vi "SAOMM-SetROIProperties.vi"(0 "PRAMMS-COMM IN":refnum<visa-resource-name>="COM4", 1 "Active Refnum":refnum<vi>, 2 "ACK Refnum":refnum<vi>, 3 "MessageType":cluster{string[], u32[]}, 11 "Error IN":errorcluster, 13 "ROIProperties":T1) -> (4 "PRAMMS-COMM OUT":refnum<visa-resource-name>="COM4", 8 "Error":bool, 15 "Error OUT":errorcluster)   [LabVIEW 2011]
panel:
  out "Array":u32[](array[numeric])
  in  "Signature":u32=1886544237
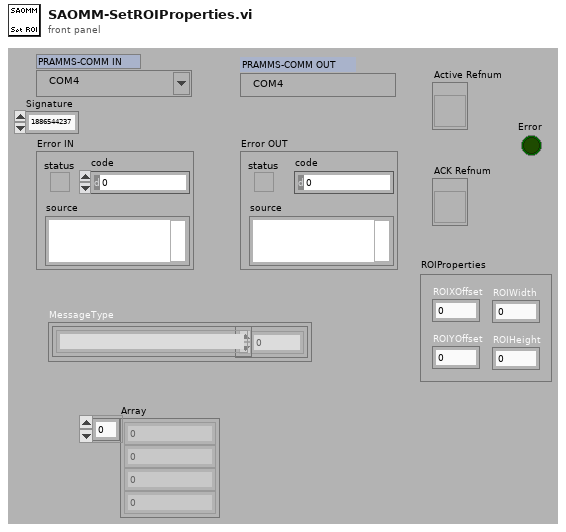
[diagram p1: front panel]
types:
  T1 = cluster{"ROIXOffset":u16, "ROIYOffset":u16, "ROIWidth":u16, "ROIHeight":u16}
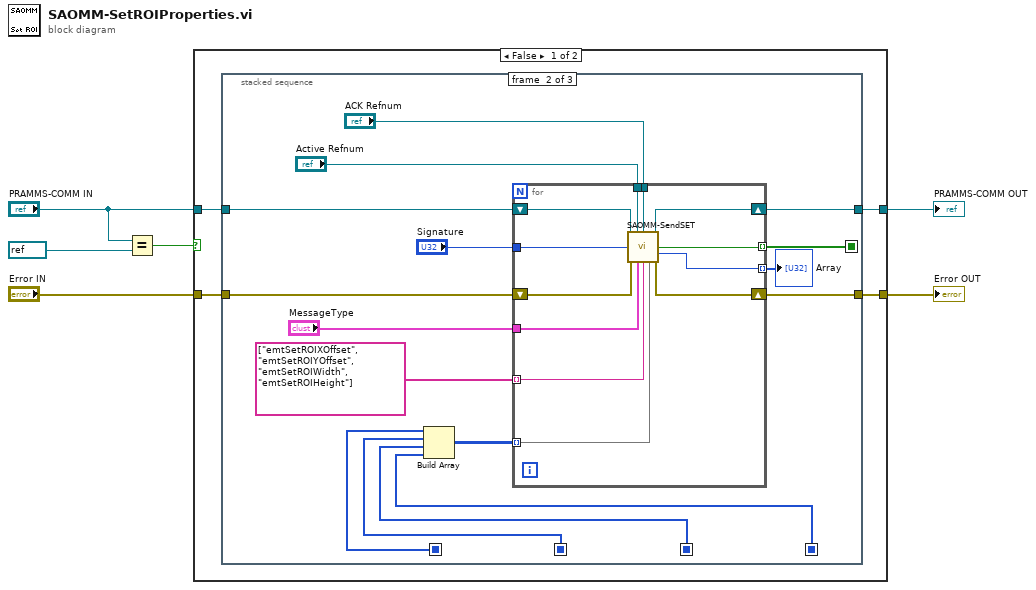
[diagram p0: block diagram]
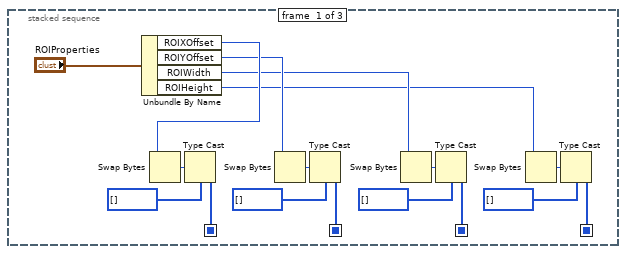
[diagram p2: hidden frame]
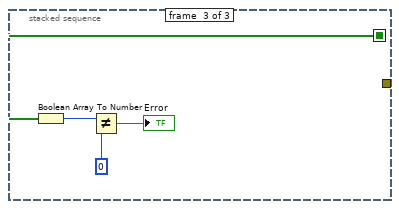
[diagram p3: hidden frame]
diagram:
  n1 = Equal?(x="PRAMMS-COMM IN", y=refnum<visa-resource-name> "-1") -> (x = y?=w5:bool)
  n2 = case shown="False" w5 {
    tunnel: "PRAMMS-COMM IN" -> [w10 w61]
    tunnel: "Error IN" -> [w9 w60]
    tunnel: [w8 w61] -> w2
    tunnel: [w7 w60] -> w1
    frame False {
      n3 = stacked-sequence {
        seq-local: [w19 _ _] -> [_ w40 _]
        seq-local: [w18 _ _] -> [_ w41 _]
        seq-local: [w17 _ _] -> [_ w42 _]
        seq-local: [w16 _ _] -> [_ w43 _]
        seq-local: [_ w31 _] -> [_ _ w59]
        tunnel: w10 -> [_ w38 _]
        tunnel: w9 -> [_ w37 _]
        tunnel: [_ w36 _] -> w8
        tunnel: [_ w35 _] -> w7
        frame #0 {
          n4 = Unbundle By Name("ROIProperties") -> ("ROIXOffset"=w14:u16, "ROIYOffset"=w13:u16, "ROIWidth"=w12:u16, "ROIHeight"=w11:u16)
          n5 = Swap Bytes(anything=w14) -> (byte swapped=w26:u16)
          n6 = Type Cast(type=u8[] [] ("Value (little endianed byte array)"), x=w26) -> (*(type *) &x=w19:u8[])
          n7 = Swap Bytes(anything=w13) -> (byte swapped=w25:u16)
          n8 = Type Cast(type=u8[] [] ("Value (little endianed byte array)"), x=w25) -> (*(type *) &x=w18:u8[])
          n9 = Swap Bytes(anything=w12) -> (byte swapped=w22:u16)
          n10 = Type Cast(type=u8[] [] ("Value (little endianed byte array)"), x=w22) -> (*(type *) &x=w17:u8[])
          n11 = Swap Bytes(anything=w11) -> (byte swapped=w21:u16)
          n12 = Type Cast(type=u8[] [] ("Value (little endianed byte array)"), x=w21) -> (*(type *) &x=w16:u8[])
        }
        frame #1 {
          n13 = Build Array(w40, w41, w42, w43) -> (w39:u8[][])
          n14 = for {
            tunnel: w39 -> [w48] mode=indexing
            shift-right: [w53] -> w36
            shift-left: w38 -> [w54]
            shift-right: [w52] -> w35
            shift-left: w37 -> [w55]
            tunnel: string[] ["emtSetROIXOffset", "emtSetROIYOffset", "emtSetROIWidth", "emtSetROIHeight"] -> [w49] mode=indexing
            tunnel: "ACK Refnum" -> [w50]
            tunnel: "Active Refnum" -> [w51]
            tunnel: [w47] -> w31 mode=indexing
            tunnel: "MessageType" -> [w46]
            tunnel: "Signature" -> [w45]
            tunnel: [w44] -> w28 mode=indexing
            n15 = call "SAOMM-SendSET.vi"("PRAMMS-COMM IN"=w54, "Active Refnum"=w51, "ACK Refnum"=w50, "Signature"=w45, "Error IN"=w55, "MessageType"=w46, "Active SET"=w49, "Value (little endianed byte array)"=w48) -> ("PRAMMS-COMM OUT"=w53:refnum<visa-resource-name>, "Error"=w47:bool, "WaitACKTime"=w44:u32, "Error OUT"=w52:errorcluster)  [unwired: 4 in]
          }
          "Array" <- w28
        }
        frame #2 {
          n16 = Boolean Array To Number(Boolean array=w59) -> (number=w58:u32)
          n17 = Not Equal?(x=w58, y=u32 0) -> (x != y?=→"Error":bool)
        }
      }
    }
    frame True {
    }
  }
  "Error OUT" <- w1
  "PRAMMS-COMM OUT" <- w2
